vi "FT10_Fornax Check Power Level.vi"(8 "Power Level in":T4, 9 "Mode in":T5, 10 "Port in":T6, 11 "JSON in":string) -> (3 "output cluster":T1)   [LabVIEW 2024]
uses:
  Controls/Control_Semi-Auto Port.ctl
  Controls/Control_Semi-Auto Mode.ctl
  Controls/Control_Semi-Auto Power Level.ctl
  Controls/Control_Semi-Auto Power Level - Change Power Cluster.ctl
  Controls/Control_Semi-Auto Power Level - For Loop Iterations.ctl
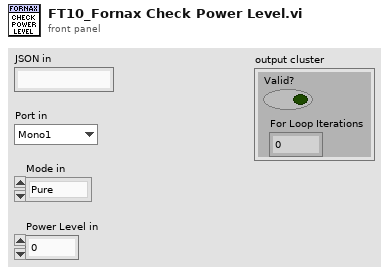
[diagram p1: front panel]
types:
  T1 = typedef "Control_Semi-Auto Power Level - Change Power Cluster.ctl" = cluster{"Valid?":T2, "For Loop Iterations":T3}
  T2 = typedef "Control_Semi-Auto Power Level - Valid" = bool
  T3 = typedef "Control_Semi-Auto Power Level - For Loop Iterations.ctl" = i32
  T4 = typedef "Control_Semi-Auto Power Level.ctl" = dbl
  T5 = typedef "Control_Semi-Auto Mode.ctl" = enum16{"Pure", "Blend", "Spray", "Fulgerate", "Standard", "Macro", "Precision", "Ligasure", "Error"}
  T6 = typedef "Control_Semi-Auto Port.ctl" = enum16{"Mono1", "Mono2", "Bipolar", "Ligasure", "Error"}
  T7 = typedef "Control_Fornax Bipolar Enum.ctl" = enum16{"Standard", "Macro", "Precision"}
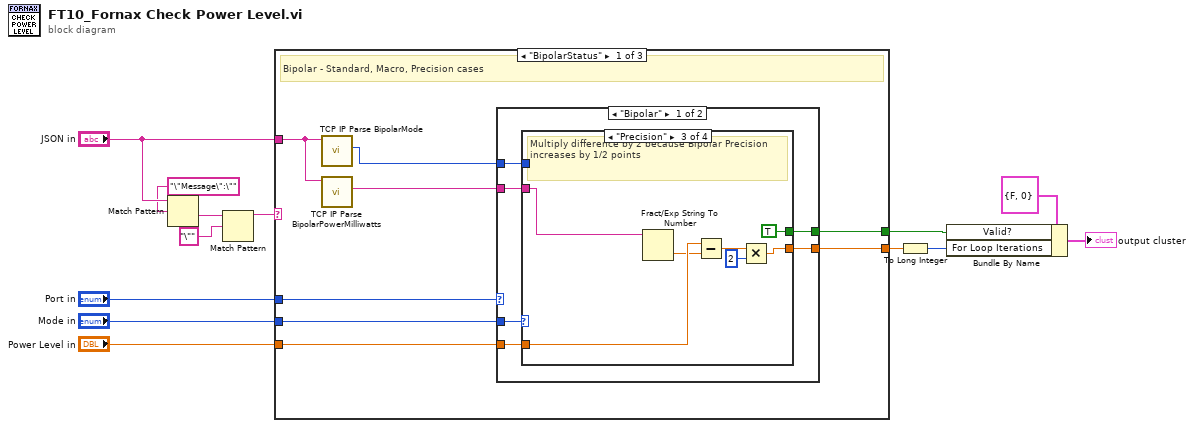
[diagram p0: block diagram]
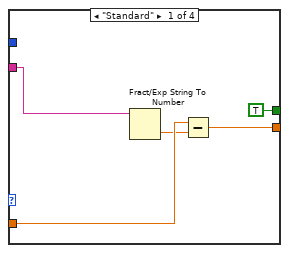
[diagram p2: hidden frame]
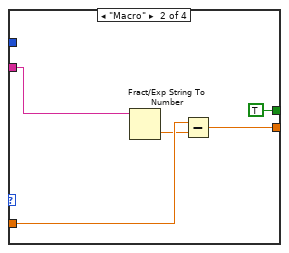
[diagram p3: hidden frame]
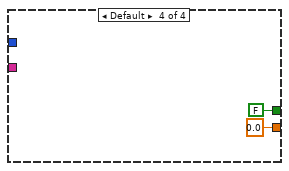
[diagram p4: hidden frame]
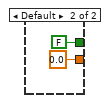
[diagram p5: hidden frame]
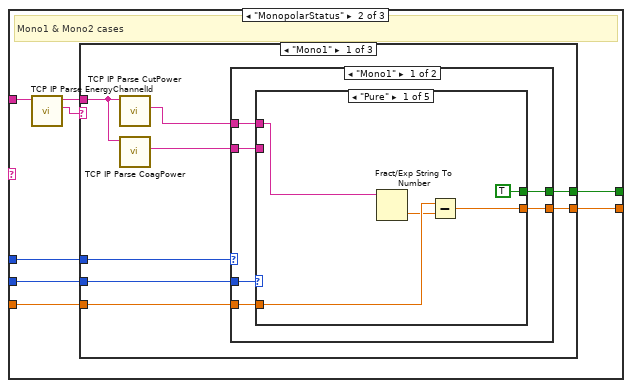
[diagram p6: hidden frame]
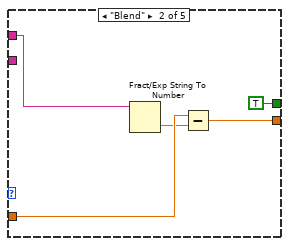
[diagram p7: hidden frame]
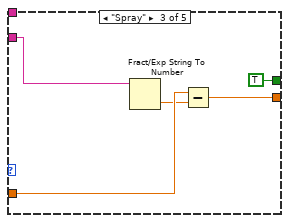
[diagram p8: hidden frame]
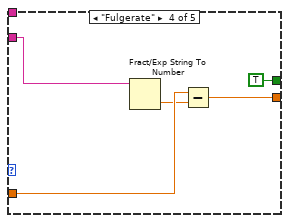
[diagram p9: hidden frame]
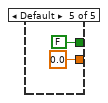
[diagram p10: hidden frame]
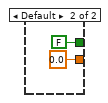
[diagram p11: hidden frame]
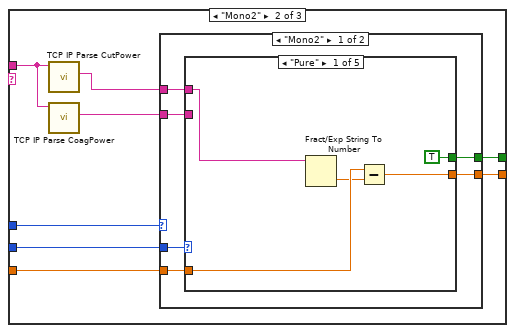
[diagram p12: hidden frame]
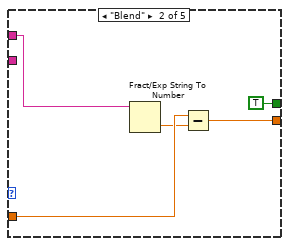
[diagram p13: hidden frame]
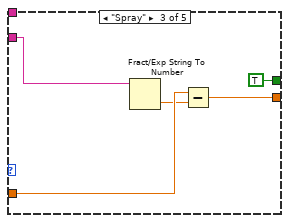
[diagram p14: hidden frame]
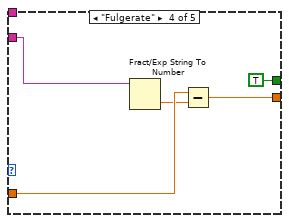
[diagram p15: hidden frame]
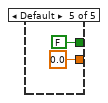
[diagram p16: hidden frame]
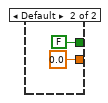
[diagram p17: hidden frame]
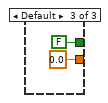
[diagram p18: hidden frame]
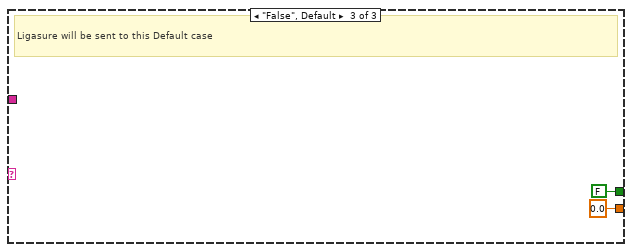
[diagram p19: hidden frame]
diagram:
  n1 = Match Pattern(string="JSON in", regular expression="\"Message\":\"") -> (after substring=w8:string)  [unwired: 1 in, 3 out]
  n2 = Match Pattern(string=w8, regular expression="\"") -> (before substring=w10:string)  [unwired: 1 in, 3 out]
  n3 = case shown="\"BipolarStatus\"" w10 {
    tunnel: "JSON in" -> [w21 w56 _]
    tunnel: "Port in" -> [w20 w53 _]
    tunnel: "Mode in" -> [w19 w52 _]
    tunnel: "Power Level in" -> [w18 w51 _]
    tunnel: [w15 w50 T4 0.0 ("Power Level in")] -> w4
    tunnel: [w14 w49 T2 FALSE ("Valid?")] -> w2
    frame "BipolarStatus" {
      # "Bipolar - Standard, Macro, Precision cases"
      n4 = call "TCP IP Parse BipolarMode.vi"("JSON in"=w21) -> ("Bipolar Enum"=w16:T7)  [unwired: 9 in, 1 out]
      n5 = call "TCP IP Parse BipolarPowerMilliwatts.vi"("JSON in"=w21) -> ("Bipolar Power (xx.x)"=w17:string)  [unwired: 9 in, 1 out]
      n6 = case shown="\"Bipolar\"" w20 {
        tunnel: w19 -> [w27 _]
        tunnel: w17 -> [w26 _]
        tunnel: w16 -> [w25 _]
        tunnel: w18 -> [w24 _]
        tunnel: [w23 T4 0.0 ("Power Level in")] -> w15
        tunnel: [w22 T2 FALSE ("Valid?")] -> w14
        frame "Bipolar" {
          n7 = case shown="\"Precision\"" w27 {
            tunnel: w26 -> [w32 w37 w44 _]
            tunnel: w25 -> [_ _ _ _]
            tunnel: w24 -> [w31 w36 w43 _]
            tunnel: [w29 w34 w39 T4 0.0 ("Power Level in")] -> w23
            tunnel: [T2 TRUE ("Valid?") T2 TRUE ("Valid?") T2 TRUE ("Valid?") T2 FALSE ("Valid?")] -> w22
            frame "Standard" {
              n8 = Fract/Exp String To Number(string=w32) -> (number=w30:dbl)  [unwired: 3 in, 1 out]
              n9 = Subtract(x=w31, y=w30) -> (x-y=w29:T4)
            }
            frame "Macro" {
              n10 = Fract/Exp String To Number(string=w37) -> (number=w35:dbl)  [unwired: 3 in, 1 out]
              n11 = Subtract(x=w36, y=w35) -> (x-y=w34:T4)
            }
            frame "Precision" {
              # "Multiply difference by 2 because Bipolar Precision increases by 1/2 points"
              n12 = Fract/Exp String To Number(string=w44) -> (number=w42:dbl)  [unwired: 3 in, 1 out]
              n13 = Subtract(x=w43, y=w42) -> (x-y=w41:T4)
              n14 = Multiply(x=w41, y=2) -> (x*y=w39:T4)
            }
            frame Default {
            }
          }
        }
        frame Default {
        }
      }
    }
    frame "MonopolarStatus" {
      # "Mono1 & Mono2 cases"
      n15 = call "TCP IP Parse EnergyChannelId.vi"("JSON in"=w56) -> ("Energy Channel ID"=w54:string, "JSON out"=w55:string)  [unwired: 9 in]
      n16 = case shown="\"Mono1\"" w54 {
        tunnel: w55 -> [w64 w102 _]
        tunnel: w53 -> [w63 w99 _]
        tunnel: w52 -> [w62 w98 _]
        tunnel: w51 -> [w59 w97 _]
        tunnel: [w58 w96 T4 0.0 ("Power Level in")] -> w50
        tunnel: [w57 w95 T2 FALSE ("Valid?")] -> w49
        frame "Mono1" {
          n17 = call "TCP IP Parse CutPower.vi"("JSON in"=w64) -> ("Cut Power"=w60:string)  [unwired: 9 in, 1 out]
          n18 = call "TCP IP Parse CoagPower.vi"("JSON in"=w64) -> ("Coag Power"=w61:string)  [unwired: 9 in, 1 out]
          n19 = case shown="\"Mono1\"" w63 {
            tunnel: w62 -> [w70 _]
            tunnel: w61 -> [w69 _]
            tunnel: w60 -> [w68 _]
            tunnel: w59 -> [w67 _]
            tunnel: [w66 T4 0.0 ("Power Level in")] -> w58
            tunnel: [w65 T2 FALSE ("Valid?")] -> w57
            frame "Mono1" {
              n20 = case shown="\"Pure\"" w70 {
                tunnel: w69 -> [_ _ w85 w90 _]
                tunnel: w68 -> [w75 w80 _ _ _]
                tunnel: w67 -> [w74 w79 w84 w89 _]
                tunnel: [w72 w77 w82 w87 T4 0.0 ("Power Level in")] -> w66
                tunnel: [T2 TRUE ("Valid?") T2 TRUE ("Valid?") T2 TRUE ("Valid?") T2 TRUE ("Valid?") T2 FALSE ("Valid?")] -> w65
                frame "Pure" {
                  n21 = Fract/Exp String To Number(string=w75) -> (number=w73:dbl)  [unwired: 3 in, 1 out]
                  n22 = Subtract(x=w74, y=w73) -> (x-y=w72:T4)
                }
                frame "Blend" {
                  n23 = Fract/Exp String To Number(string=w80) -> (number=w78:dbl)  [unwired: 3 in, 1 out]
                  n24 = Subtract(x=w79, y=w78) -> (x-y=w77:T4)
                }
                frame "Spray" {
                  n25 = Fract/Exp String To Number(string=w85) -> (number=w83:dbl)  [unwired: 3 in, 1 out]
                  n26 = Subtract(x=w84, y=w83) -> (x-y=w82:T4)
                }
                frame "Fulgerate" {
                  n27 = Fract/Exp String To Number(string=w90) -> (number=w88:dbl)  [unwired: 3 in, 1 out]
                  n28 = Subtract(x=w89, y=w88) -> (x-y=w87:T4)
                }
                frame Default {
                }
              }
            }
            frame Default {
            }
          }
        }
        frame "Mono2" {
          n29 = call "TCP IP Parse CutPower.vi"("JSON in"=w102) -> ("Cut Power"=w101:string)  [unwired: 9 in, 1 out]
          n30 = call "TCP IP Parse CoagPower.vi"("JSON in"=w102) -> ("Coag Power"=w100:string)  [unwired: 9 in, 1 out]
          n31 = case shown="\"Mono2\"" w99 {
            tunnel: w98 -> [w108 _]
            tunnel: w100 -> [w107 _]
            tunnel: w101 -> [w106 _]
            tunnel: w97 -> [w105 _]
            tunnel: [w104 T4 0.0 ("Power Level in")] -> w96
            tunnel: [w103 T2 FALSE ("Valid?")] -> w95
            frame "Mono2" {
              n32 = case shown="\"Pure\"" w108 {
                tunnel: w107 -> [_ _ w123 w128 _]
                tunnel: w106 -> [w113 w118 _ _ _]
                tunnel: w105 -> [w112 w117 w122 w127 _]
                tunnel: [w110 w115 w120 w125 T4 0.0 ("Power Level in")] -> w104
                tunnel: [T2 TRUE ("Valid?") T2 TRUE ("Valid?") T2 TRUE ("Valid?") T2 TRUE ("Valid?") T2 FALSE ("Valid?")] -> w103
                frame "Pure" {
                  n33 = Fract/Exp String To Number(string=w113) -> (number=w111:dbl)  [unwired: 3 in, 1 out]
                  n34 = Subtract(x=w112, y=w111) -> (x-y=w110:T4)
                }
                frame "Blend" {
                  n35 = Fract/Exp String To Number(string=w118) -> (number=w116:dbl)  [unwired: 3 in, 1 out]
                  n36 = Subtract(x=w117, y=w116) -> (x-y=w115:T4)
                }
                frame "Spray" {
                  n37 = Fract/Exp String To Number(string=w123) -> (number=w121:dbl)  [unwired: 3 in, 1 out]
                  n38 = Subtract(x=w122, y=w121) -> (x-y=w120:T4)
                }
                frame "Fulgerate" {
                  n39 = Fract/Exp String To Number(string=w128) -> (number=w126:dbl)  [unwired: 3 in, 1 out]
                  n40 = Subtract(x=w127, y=w126) -> (x-y=w125:T4)
                }
                frame Default {
                }
              }
            }
            frame Default {
            }
          }
        }
        frame Default {
        }
      }
    }
    frame "False", Default {
      # "Ligasure will be sent to this Default case"
    }
  }
  n41 = To Long Integer(number=w4) -> (32bit integer=w3:i32)
  n42 = Bundle By Name(cluster=T1 {"Valid?"=FALSE, "For Loop Iterations"=0}, "Valid?"=w2, "For Loop Iterations"=w3) -> (→"output cluster":T1)
